vi "Pause.vi"(8 "error in (no error)":errorcluster, 11 "State in":T1={"State"=enum."Idle", "Start Time"=timestamp(0 s since 1904-01-01), "Configuration"={"Cycle Period"=0.0, "Setpoint Entry"=0.0, "Output Device"=enum."Huber Ministat 230", "Huber Ministat 230 Settings"={"VISA resource name"="", "Simulated?"=FALSE}, "Lauda Settings"={"VISA resource name"="", "Simulated?"=FALSE, "Pump Power"=2}, "Julabo FP-50 Settings"={"VISA resource name"="", "Simulated?"=FALSE, "Pump Power"=2}, "Internal Control?"=FALSE, "Huber Unistat 410 Settings"={"VISA resource name"="", "Simulated?"=FALSE}}, "Current Time"=timestamp(0 s since 1904-01-01), "First Iteration"=FALSE, "Data"={"TCU Speed"=0.0, "Temperature"=0.0}, "Process Name"="", "TCU On?"=FALSE, "Output Error"=FALSE, "Start Log"=FALSE, "Power Level Changed"=FALSE} {"Configuration"."Julabo FP-50 Settings"."Pump Power" min=0 max=8 step=1; "Configuration"."Lauda Settings"."Pump Power" min=0 max=8 step=1}) -> (0 "error out":errorcluster, 3 "State out":T1={"State"=enum."Idle", "Start Time"=timestamp(0 s since 1904-01-01), "Configuration"={"Cycle Period"=0.0, "Setpoint Entry"=0.0, "Output Device"=enum."Huber Ministat 230", "Huber Ministat 230 Settings"={"VISA resource name"="", "Simulated?"=FALSE}, "Lauda Settings"={"VISA resource name"="", "Simulated?"=FALSE, "Pump Power"=2}, "Julabo FP-50 Settings"={"VISA resource name"="", "Simulated?"=FALSE, "Pump Power"=2}, "Internal Control?"=FALSE, "Huber Unistat 410 Settings"={"VISA resource name"="", "Simulated?"=FALSE}}, "Current Time"=timestamp(0 s since 1904-01-01), "First Iteration"=FALSE, "Data"={"TCU Speed"=0.0, "Temperature"=0.0}, "Process Name"="", "TCU On?"=FALSE, "Output Error"=FALSE, "Start Log"=FALSE, "Power Level Changed"=FALSE} {"Configuration"."Julabo FP-50 Settings"."Pump Power" min=0 max=8 step=1; "Configuration"."Lauda Settings"."Pump Power" min=0 max=8 step=1})   [LabVIEW 2018, in "TCU Module.lvlib" / "TCU Module Engine.lvlib"]
uses:
  TCU Module Engine.lvlib
  TCU State Cluster.ctl
  State Enum.ctl
  TCU Module Settings Cluster.ctl
  Output Devices.ctl
  Huber TCU/Huber Settings.ctl
  Lauda Integral XT-150 TCU/Lauda Settings.ctl
  Julabo Type 1 TCU/Julabo Type 1 TCU Folder/Julabo FP-50 Settings.ctl
  Huber Unistat 410 TCU/Huber Unistat 410 Settings.ctl
  Huber TCU/Huber Ministat 230 TCU.lvlib
  Lauda Integral XT-150 TCU/Lauda TCU.lvlib
  Julabo Type 1 TCU/Julabo Type 1 TCU Folder/Julabo Type FP-50 TCU.lvlib
  Huber Unistat 410 TCU/Huber Unistat 410 TCU.lvlib
  TCU Module.lvlib
panel:
  # "Output Instruments"
  # "Output Instruments"
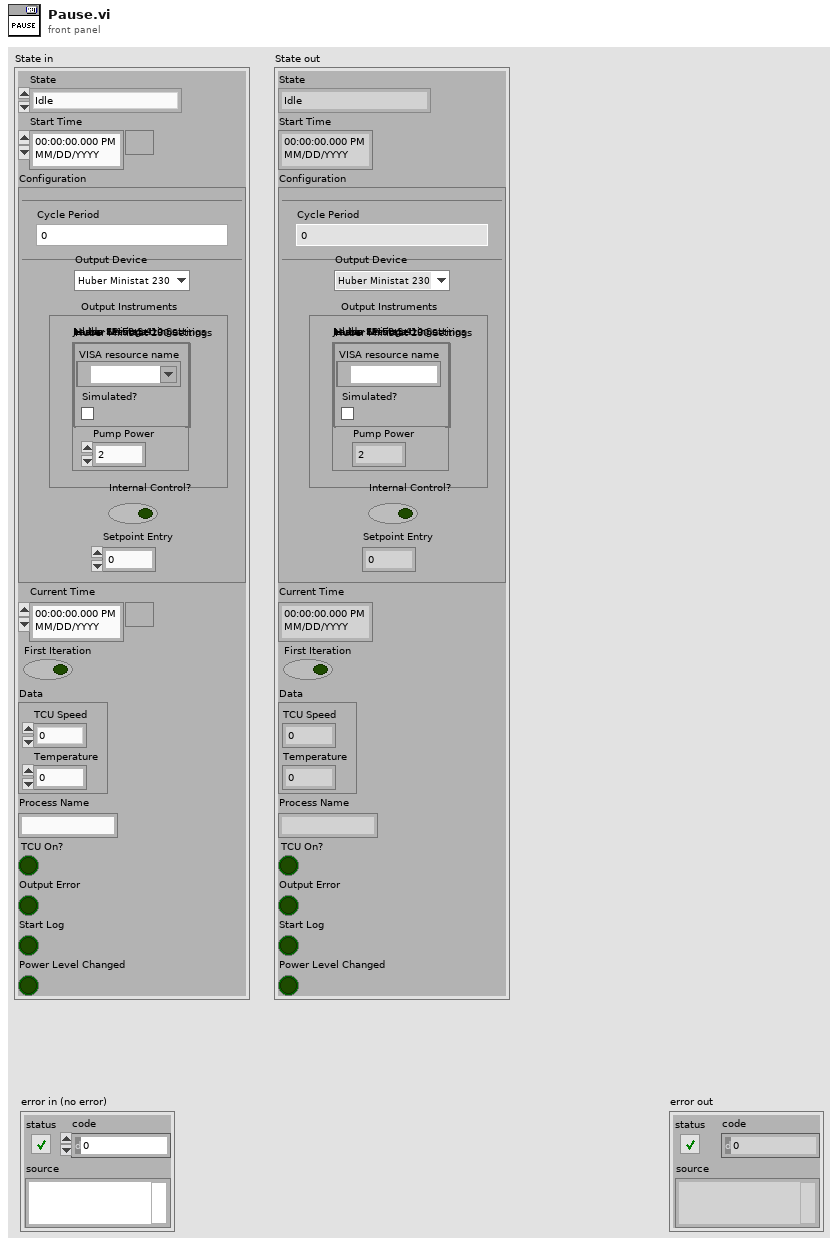
[diagram p1: front panel]
types:
  T1 = typedef "TCU Module.lvlib/TCU Module Engine.lvlib/TCU State Cluster.ctl" = cluster{"State":T2, "Start Time":timestamp, "Configuration":T3, "Current Time":timestamp, "First Iteration":bool, "Data":cluster{"TCU Speed":dbl, "Temperature":dbl}, "Process Name":string, "TCU On?":bool, "Output Error":bool, "Start Log":bool, "Power Level Changed":bool}
  T2 = typedef "TCU Module.lvlib/TCU Module Engine.lvlib/State Enum.ctl" = enum16{"Measuring", "Idle", "Paused"}
  T3 = typedef "TCU Module.lvlib/TCU Module Settings Cluster.ctl" = cluster{"Cycle Period":dbl, "Setpoint Entry":dbl, "Output Device":T4, "Huber Ministat 230 Settings":T5, "Lauda Settings":T6, "Julabo FP-50 Settings":T7, "Internal Control?":bool, "Huber Unistat 410 Settings":T8}
  T4 = typedef "Output Devices.ctl" = enum16{"Default", "Huber Ministat 230", "Huber Unistat 410", "Lauda XT-150", "Julabo FP-50"}
  T5 = typedef "Huber Ministat 230 TCU.lvlib/Huber Settings.ctl" = cluster{"VISA resource name":refnum<visa-resource-name>, "Simulated?":bool}
  T6 = typedef "Lauda TCU.lvlib/Lauda Settings.ctl" = cluster{"VISA resource name":refnum<visa-resource-name>, "Simulated?":bool, "Pump Power":i32}
  T7 = typedef "Julabo Type FP-50 TCU.lvlib/Julabo FP-50 Settings.ctl" = cluster{"VISA resource name":refnum<visa-resource-name>, "Simulated?":bool, "Pump Power":i32}
  T8 = typedef "Huber Unistat 410 TCU.lvlib/Huber Unistat 410 Settings.ctl" = cluster{"VISA resource name":refnum<visa-resource-name>, "Simulated?":bool}
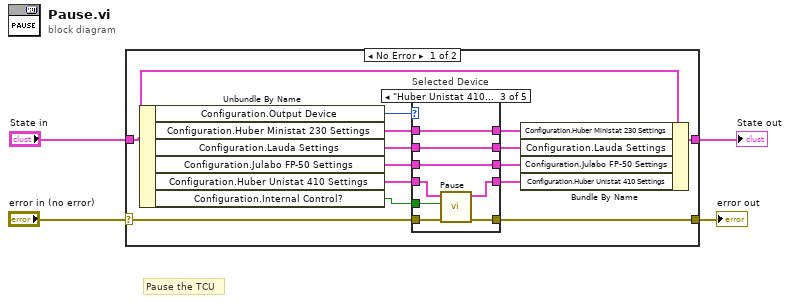
[diagram p0: block diagram]
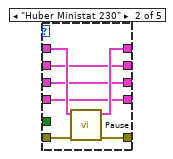
[diagram p3: hidden frame]
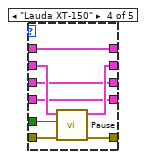
[diagram p4: hidden frame]
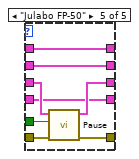
[diagram p5: hidden frame]
diagram:
  # "Pause the TCU"
  n1 = case shown="No Error" "error in (no error)" {
    selector: "error in (no error)" -> [w15 w56]
    tunnel: [w16 w56] -> w3
    tunnel: "State in" -> [w18 w55]
    tunnel: [w17 w55] -> w1
    frame No Error {
      n2 = Unbundle By Name(w18) -> ("Configuration.Output Device"=w14:T4, "Configuration.Huber Ministat 230 Settings"=w13:T5, "Configuration.Lauda Settings"=w11:T6, "Configuration.Julabo FP-50 Settings"=w8:T7, "Configuration.Huber Unistat 410 Settings"=w7:T8, "Configuration.Internal Control?"=w5:bool)
      n3 = case "Selected Device" shown="\"Huber Unistat 410\"" w14 {
        tunnel: [w23 w30 w32 w45 w51] -> w16
        tunnel: w15 -> [w23 w29 w33 w46 w52]
        tunnel: w13 -> [w22 w28 w38 w42 w54]
        tunnel: [w22 w27 w38 w42 w54] -> w12
        tunnel: w11 -> [w21 w26 w37 w43 w53]
        tunnel: [w21 w26 w37 w44 w53] -> w10
        tunnel: [w20 w25 w36 w41 w49] -> w9
        tunnel: w8 -> [w20 w25 w36 w41 w50]
        tunnel: w7 -> [w19 w24 w35 w40 w47]
        tunnel: [w19 w24 w34 w40 w47] -> w6
        tunnel: w5 -> [_ _ w31 w39 w48]
        frame "Default", Default {
        }
        frame "Huber Ministat 230" {
          n4 = call "Pause.vi"("error in (no error)"=w29, "Huber Settings"=w28) -> ("error out"=w30:errorcluster, "Huber Settings"=w27:T5)  [unwired: 8 in]
        }
        frame "Huber Unistat 410" {
          n5 = call "Pause.vi"("error in (no error)"=w33, "Internal?"=w31, "Huber Settings"=w35) -> ("error out"=w32:errorcluster, "Huber Settings"=w34:T8)  [unwired: 7 in]
        }
        frame "Lauda XT-150" {
          n6 = call "Pause.vi"("error in (no error)"=w46, "Internal?"=w39, "Huber Settings"=w43) -> ("error out"=w45:errorcluster, "Huber Settings"=w44:T6)  [unwired: 7 in]
        }
        frame "Julabo FP-50" {
          n7 = call "Pause.vi"("error in (no error)"=w52, "Internal?"=w48, "Julabo FP-50 Settings"=w50) -> ("error out"=w51:errorcluster, "Julabo FP-50 Settings"=w49:T7)  [unwired: 7 in]
        }
      }
      n8 = Bundle By Name(cluster=w18, "Configuration.Huber Ministat 230 Settings"=w12, "Configuration.Lauda Settings"=w10, "Configuration.Julabo FP-50 Settings"=w9, "Configuration.Huber Unistat 410 Settings"=w6) -> (w17:T1)
    }
    frame Error {
    }
  }
  "error out" <- w3
  "State out" <- w1
